vi "Close Interface.vi"(8 "error in (no error)":errorcluster, 11 "CAN Frame Sessions":T1={"Session_Control"="Session_Control", "Session_Params"="Session_Params", "Session_Actuals"="Session_Actuals", "Session_Acknowledge"="Session_Acknowledge", "Session_H2_Sensor"="H2_Sensor_Session"}) -> (0 "error out":errorcluster)   [LabVIEW 2025, in "phlair-busch-can-bus.lvlib"]
uses:
  phlair-busch-can-bus.lvlib
  CAN Frame Sessions.ctl
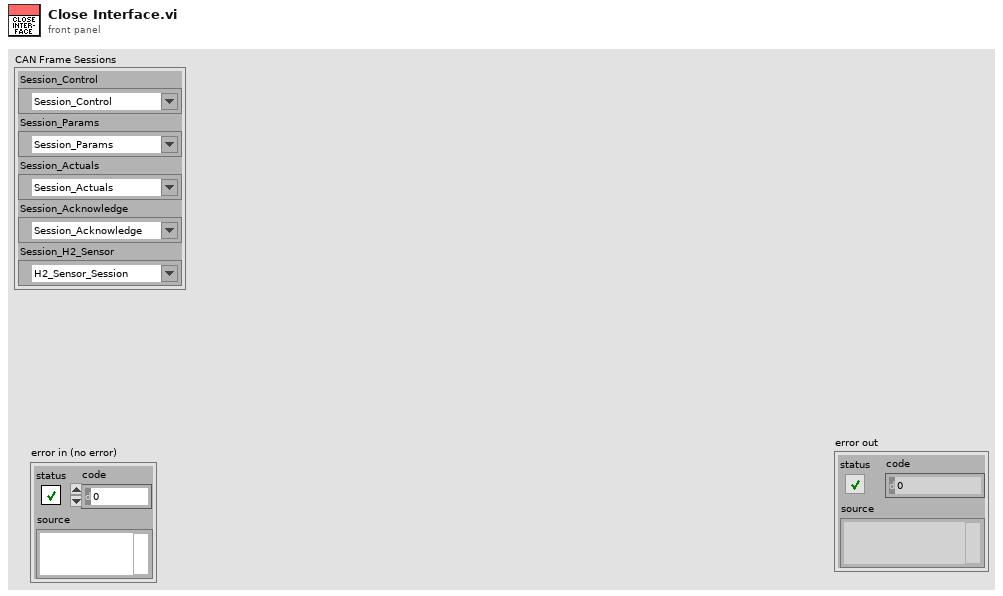
[diagram p1: front panel]
types:
  T1 = typedef "phlair-busch-can-bus.lvlib/CAN Frame Sessions.ctl" = cluster{"Session_Control":refnum<k21>, "Session_Params":refnum<k21>, "Session_Actuals":refnum<k21>, "Session_Acknowledge":refnum<k21>, "Session_H2_Sensor":refnum<k21>}
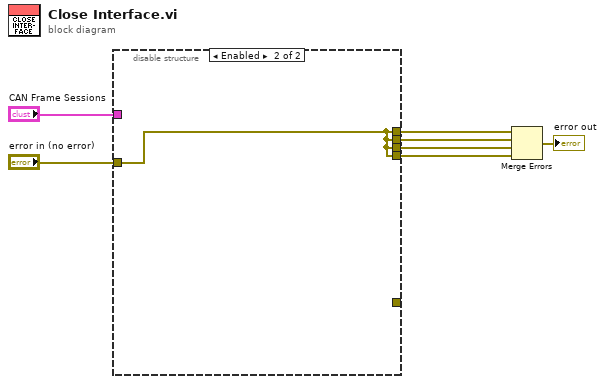
[diagram p0: block diagram]
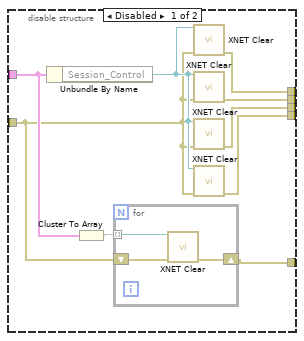
[diagram p2: hidden frame]
diagram:
  n1 = disable-structure shown="Enabled" {
    disable-tunnel: "CAN Frame Sessions" -> [w10 _]
    disable-tunnel: [w15 w20] -> w7
    disable-tunnel: [w14 w20] -> w6
    disable-tunnel: [w13 w20] -> w5
    disable-tunnel: [w12 w20] -> w4
    disable-tunnel: "error in (no error)" -> [w9 w20]
    disable-tunnel: [w8 _] -> _
    frame Disabled {
      n2 = Unbundle By Name(w10) -> ("Session_Control"=w16:refnum<k21>)
      n3 = Cluster To Array(cluster=w10) -> (array=w11:refnum<k21>[])
      n4 = for {
        tunnel: w11 -> [w19] mode=indexing
        shift-right: [w18] -> w8
        shift-left: w9 -> [w17]
        n5 = call <vilib>:"XNET Clear.vi"("session in"=w19, "error in (no error)"=w17) -> ("error out"=w18:errorcluster)  [unwired: 13 in]
      }
      n6 = call <vilib>:"XNET Clear.vi"("session in"=w16, "error in (no error)"=w9) -> ("error out"=w15:errorcluster)  [unwired: 13 in]
      n7 = call <vilib>:"XNET Clear.vi"("session in"=w16, "error in (no error)"=w9) -> ("error out"=w14:errorcluster)  [unwired: 13 in]
      n8 = call <vilib>:"XNET Clear.vi"("session in"=w16, "error in (no error)"=w9) -> ("error out"=w13:errorcluster)  [unwired: 13 in]
      n9 = call <vilib>:"XNET Clear.vi"("session in"=w16, "error in (no error)"=w9) -> ("error out"=w12:errorcluster)  [unwired: 13 in]
    }
    frame Enabled {
    }
  }
  n10 = Merge Errors(w7, w6, w5, w4) -> (→"error out":errorcluster)
